vi "Abort VI.vi"() -> ()   [LabVIEW 2017]
panel:
  in  "Cancel":bool
  in  "Abort":bool
  in  "Running VIs":u16(ring) items=["Main.vi"]
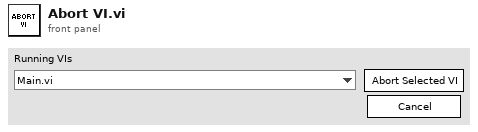
[diagram p1: front panel]
types:
  T1 = enum32{"Bad", "Idle", "Run top level", "Running"}
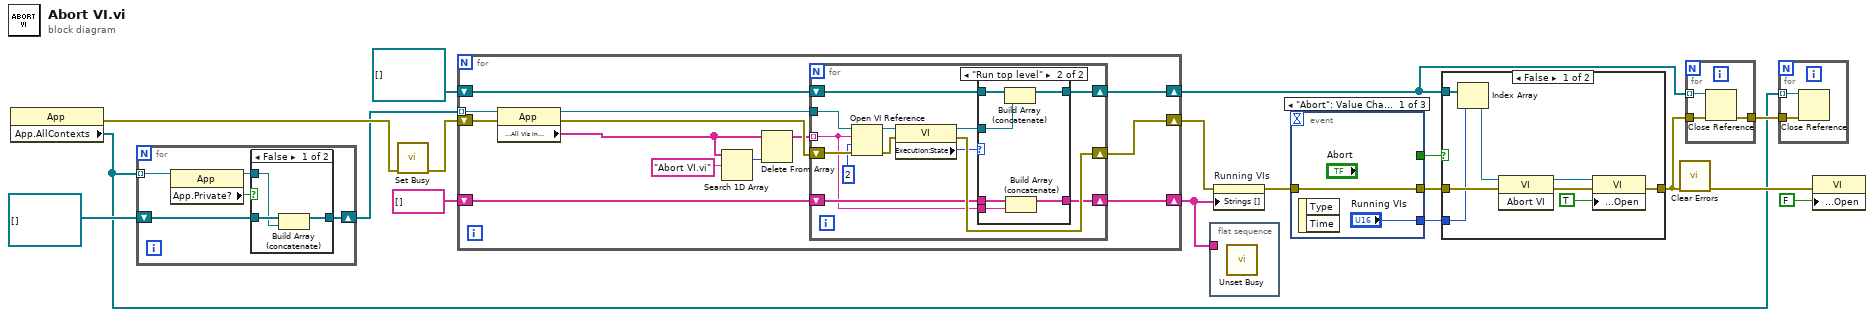
[diagram p0: block diagram]
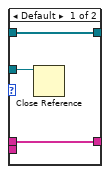
[diagram p3: hidden frame]
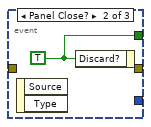
[diagram p5: hidden frame]
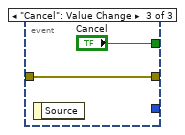
[diagram p6: hidden frame]
diagram:
  n1 = property class="App"() -> (error out=w9:errorcluster, "App.AllContexts"=w2:refnum<vi>[])  [unwired: 2 in, 1 out]
  n2 = for {
    tunnel: w2 -> [w23] mode=indexing
    shift-right: [w20] -> w1
    shift-left: refnum<vi>[] [] ("Application:All Contexts") -> [w21]
    n3 = property class="App"(reference=w23) -> (reference out=w19:refnum<vi>, "App.Private?"=w22:bool)  [unwired: 1 in, 1 out]
    n4 = case shown="False" w22 {
      tunnel: w21 -> [w26 w27]
      tunnel: [w24 w27] -> w20
      tunnel: w19 -> [w25 _]
      frame False {
        n5 = Build Array (concatenate)(w26, w25) -> (w24:refnum<vi>[])
      }
      frame True {
      }
    }
  }
  n6 = call <vilib>:"Set Busy.vi"("error in (no error)"=w9) -> ("error out"=w8:errorcluster)  [unwired: 3 in, 7 out]
  n7 = for {
    tunnel: w1 -> [w34] mode=indexing
    shift-right: [w33] -> w12
    shift-left: refnum<vi>[] [] -> [w32]
    shift-right: [w30] -> w7
    shift-left: string[] [] ("Application:All System VIs in Memory") -> [w31]
    shift-right: [w39] -> w18
    shift-left: w8 -> [w35]
    n8 = property class="App"(reference=w34, error in=w35) -> (reference out=w29:refnum<vi>, error out=w40:errorcluster, "Application:All VIs In Memory"=w28:string[])
    n9 = Search 1D Array(1D array=w28, element="Abort VI.vi") -> (index of element=w36:i32)  [unwired: 1 out]
    n10 = Delete From Array(array=w28, index=w36) -> (array with subset deleted=w37:string[])  [unwired: 1 in, 1 out]
    n11 = for {
      shift-right: [w50] -> w39
      shift-left: w40 -> [w53]
      tunnel: w37 -> [w43] mode=indexing
      shift-right: [w47] -> w33
      shift-left: w32 -> [w48]
      shift-right: [w45] -> w30
      shift-left: w31 -> [w46]
      tunnel: w29 -> [w42]
      n12 = Open VI Reference(application reference (local)=w42, vi path=w43, options=2, error in (no error)=w53) -> (vi reference=w52:refnum<vi>, error out=w51:errorcluster)  [unwired: 2 out]
      n13 = property class="VI"(reference=w52, error in=w51) -> (reference out=w44:refnum<vi>, error out=w50:errorcluster, "Execution:State"=w49:T1)
      n14 = case shown="\"Run top level\"" w49 {
        tunnel: w48 -> [w56 w62]
        tunnel: [w56 w61] -> w47
        tunnel: [w55 w58] -> w45
        tunnel: w46 -> [w55 w59]
        tunnel: w44 -> [w54 w60]
        tunnel: w43 -> [_ w57]
        frame Default {
          n15 = Close Reference(reference=w54) -> ()  [unwired: 1 in, 1 out]
        }
        frame "Run top level" {
          n16 = Build Array (concatenate)(w62, w60) -> (w61:refnum<vi>[])
          n17 = Build Array (concatenate)(w59, w57) -> (w58:string[])
        }
      }
    }
  }
  n18 = flat-sequence {
    tunnel: w7 -> [_]
    frame #0 {
      n19 = call <vilib>:"Unset Busy.vi"() -> ()  [unwired: 2 in, 10 out]
    }
  }
  n20 = property on="Running VIs" class="Ring (strict)"(error in=w18, "Strings []"=w7) -> (error out=w17:errorcluster)  [unwired: 1 in, 1 out]
  n21 = event shown="[0] \"Abort\": Value Change" {
    selector: _ -> [_ _ _]
    dyn-events: _ -> [_ _ _]
    timeout: _ -> [_ _ _]
    tunnel: w17 -> [w63 _ w66]
    tunnel: [_ w65 "Cancel"] -> w16
    tunnel: ["Running VIs" _ _] -> w14
    tunnel: [w63 _ w66] -> w15
    event "Abort": Value Change {
      n22 = event-data() -> ()  [unwired: 3 out]
    }
    event Panel Close? {
      w65 = TRUE ("Discard?")
      n23 = event-data() -> ()  [unwired: 3 out]
      n24 = event-data("Discard?"=w65) -> ()  [unwired: 1 in, 1 out]
    }
    event "Cancel": Value Change {
      n25 = event-data() -> ()  [unwired: 2 out]
    }
  }
  n26 = case shown="False" w16 {
    tunnel: w15 -> [w72 w76]
    tunnel: w14 -> [w70 _]
    tunnel: w12 -> [w71 _]
    tunnel: [w68 w76] -> w6
    frame False {
      n27 = Index Array(array=w71, index=w70) -> (element=w69:refnum<vi>)
      n28 = invoke class="VI" method="Abort VI"(reference=w69, error in=w72) -> (reference out=w75:refnum<vi>, error out=w74:errorcluster)  [unwired: 1 in, 1 out]
      n29 = property class="VI"(reference=w75, error in=w74, "Front Panel Window:Open"=TRUE) -> (error out=w68:errorcluster)  [unwired: 1 out]
    }
    frame True {
    }
  }
  n30 = call <vilib>:"Clear Errors.vi"("error in (no error)"=w6) -> ("error out"=w5:errorcluster)  [unwired: 1 in, 5 out]
  n31 = for {
    tunnel: w12 -> [w79] mode=indexing
    tunnel: w6 -> [w78]
    tunnel: [w77] -> w3
    n32 = Close Reference(reference=w79, error in (no error)=w78) -> (error out=w77:errorcluster)
  }
  n33 = for {
    tunnel: w2 -> [w81] mode=indexing
    tunnel: w3 -> [w80]
    n34 = Close Reference(reference=w81, error in (no error)=w80) -> ()  [unwired: 1 out]
  }
  n35 = property class="VI"(error in=w5, "Front Panel Window:Open"=FALSE) -> ()  [unwired: 1 in, 2 out]
